vi "FTW-Test-JSON-Path.vi"() -> (0 "Test Result":errorcluster)   [LabVIEW 2015]
uses:
  src/json/FTW-JSON-Type.ctl
  src/json/core/FTW-JSON-Core-Type.ctl
  src/reflection/FTW-Reflection-Types.ctl
  src/json/core/FTW-JSON-Core-NumericType.vi
  lib/FTW-KernelFilepath.vi
  src/error/FTW-ERR-ThrowError.vi
  src/error/FTW-ERR-ThrowInvalidReferenceError.vi
  src/json/core/FTW-JSON-Core-ElementType.vi
  codegen/xnode/json/fetch/FTW-JSON-Core-GetFlattenedValue.vi
  codegen/xnode/FTW-JSON-Fetch.xnode
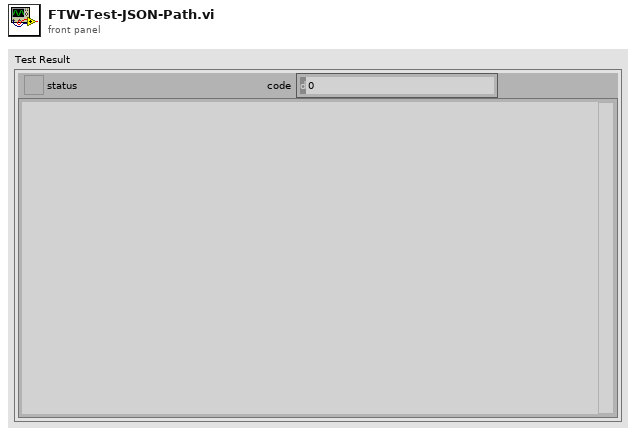
[diagram p1: front panel]
types:
  T1 = typedef "FTW-JSON-Type.ctl" = enum8{"Not Found", "Object", "Array", "String", "Number", "Boolean", "null"}
  T2 = cluster{"Path":string, "ExpectedValue":i32, "ExpectedType":T1}[]
  T3 = typedef "FTW-Type-JSON.ctl" = refnum<data-value>
  T4 = typedef "FTW-JSON-Core-Type.ctl" = enum8{"Object", "Array", "String", "Integer", "Floating Point", "true", "false", "null", "undefined"}
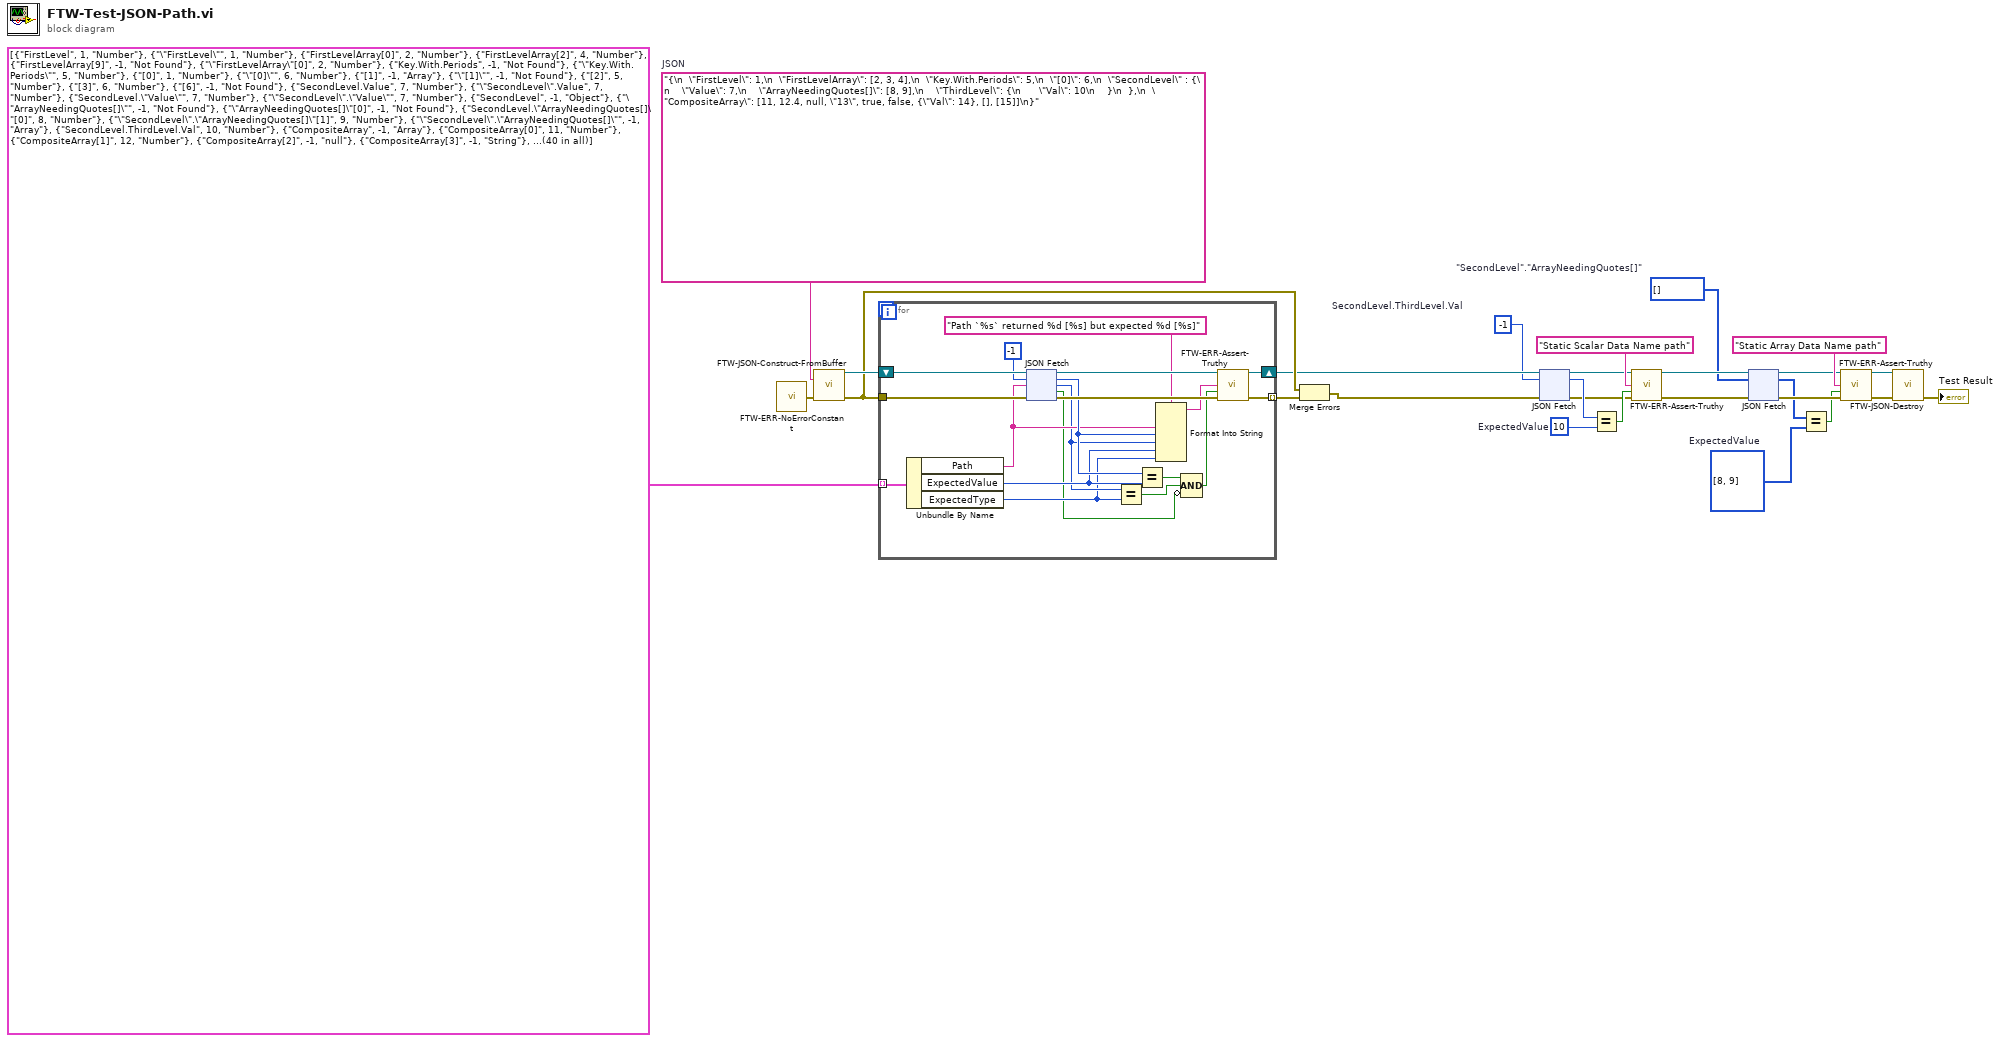
[diagram p0: block diagram]
diagram:
  w4 = i32[] [8, 9]  # ExpectedValue
  w2 = i32[] []  # "SecondLevel"."ArrayNeedingQuotes[]"
  w13 = 10  # ExpectedValue
  w3 = -1  # SecondLevel.ThirdLevel.Val
  w24 = "{\n  \"FirstLevel\": 1,\n  \"FirstLevelArray\": [2, 3, 4],\n  \"Key.With.Periods\": 5,\n  \"[0]\": 6,\n  \"SecondLevel\" : {\n    \"Value\": 7,\n    \"ArrayNeedingQuotes[]\": [8, 9],\n    \"ThirdLevel\": {\n      \"Val\": 10\n    }\n  },\n  \"CompositeArray\": [11, 12.4, null, \"13\", true, false, {\"Val\": 14}, [], [15]]\n}"  # JSON
  n1 = call "FTW-ERR-NoErrorConstant.vi"() -> ("no error"=w25:errorcluster)
  n2 = call "FTW-JSON-Construct-FromBuffer.vi"("JSON String (UTF-8)"=w24, "error in"=w25) -> ("JSON"=w23:T3, "error out"=w22:errorcluster)  [unwired: 12 in]
  n3 = for {
    tunnel: w22 -> [w43]
    tunnel: T2 [{"Path"="FirstLevel", "ExpectedValue"=1, "ExpectedType"=enum."Number"}, {"Path"="\"FirstLevel\"", "ExpectedValue"=1, "ExpectedType"=enum."Number"}, {"Path"="FirstLevelArray[0]", "ExpectedValue"=2, "ExpectedType"=enum."Number"}, {"Path"="FirstLevelArray[2]", "ExpectedValue"=4, "ExpectedType"=enum."Number"}, {"Path"="FirstLevelArray[9]", "ExpectedValue"=-1, "ExpectedType"=enum."Not Found"}, {"Path"="\"FirstLevelArray\"[0]", "ExpectedValue"=2, "ExpectedType"=enum."Number"}, {"Path"="Key.With.Periods", "ExpectedValue"=-1, "ExpectedType"=enum."Not Found"}, {"Path"="\"Key.With.Periods\"", "ExpectedValue"=5, "ExpectedType"=enum."Number"}, {"Path"="[0]", "ExpectedValue"=1, "ExpectedType"=enum."Number"}, {"Path"="\"[0]\"", "ExpectedValue"=6, "ExpectedType"=enum."Number"}, {"Path"="[1]", "ExpectedValue"=-1, "ExpectedType"=enum."Array"}, {"Path"="\"[1]\"", "ExpectedValue"=-1, "ExpectedType"=enum."Not Found"}, {"Path"="[2]", "ExpectedValue"=5, "ExpectedType"=enum."Number"}, {"Path"="[3]", "ExpectedValue"=6, "ExpectedType"=enum."Number"}, {"Path"="[6]", "ExpectedValue"=-1, "ExpectedType"=enum."Not Found"}, {"Path"="SecondLevel.Value", "ExpectedValue"=7, "ExpectedType"=enum."Number"}, {"Path"="\"SecondLevel\".Value", "ExpectedValue"=7, "ExpectedType"=enum."Number"}, {"Path"="SecondLevel.\"Value\"", "ExpectedValue"=7, "ExpectedType"=enum."Number"}, {"Path"="\"SecondLevel\".\"Value\"", "ExpectedValue"=7, "ExpectedType"=enum."Number"}, {"Path"="SecondLevel", "ExpectedValue"=-1, "ExpectedType"=enum."Object"}, {"Path"="\"ArrayNeedingQuotes[]\"", "ExpectedValue"=-1, "ExpectedType"=enum."Not Found"}, {"Path"="\"ArrayNeedingQuotes[]\"[0]", "ExpectedValue"=-1, "ExpectedType"=enum."Not Found"}, {"Path"="SecondLevel.\"ArrayNeedingQuotes[]\"[0]", "ExpectedValue"=8, "ExpectedType"=enum."Number"}, {"Path"="\"SecondLevel\".\"ArrayNeedingQuotes[]\"[1]", "ExpectedValue"=9, "ExpectedType"=enum."Number"}, {"Path"="\"SecondLevel\".\"ArrayNeedingQuotes[]\"", "ExpectedValue"=-1, "ExpectedType"=enum."Array"}, {"Path"="SecondLevel.ThirdLevel.Val", "ExpectedValue"=10, "ExpectedType"=enum."Number"}, {"Path"="CompositeArray", "ExpectedValue"=-1, "ExpectedType"=enum."Array"}, {"Path"="CompositeArray[0]", "ExpectedValue"=11, "ExpectedType"=enum."Number"}, {"Path"="CompositeArray[1]", "ExpectedValue"=12, "ExpectedType"=enum."Number"}, {"Path"="CompositeArray[2]", "ExpectedValue"=-1, "ExpectedType"=enum."null"}, {"Path"="CompositeArray[3]", "ExpectedValue"=-1, "ExpectedType"=enum."String"}, {"Path"="CompositeArray[4]", "ExpectedValue"=1, "ExpectedType"=enum."Boolean"}, {"Path"="CompositeArray[5]", "ExpectedValue"=0, "ExpectedType"=enum."Boolean"}, {"Path"="CompositeArray[6]", "ExpectedValue"=-1, "ExpectedType"=enum."Object"}, {"Path"="CompositeArray[6].Val", "ExpectedValue"=14, "ExpectedType"=enum."Number"}, {"Path"="CompositeArray[7]", "ExpectedValue"=-1, "ExpectedType"=enum."Array"}, {"Path"="CompositeArray[8][0]", "ExpectedValue"=15, "ExpectedType"=enum."Number"}, {"Path"="CompositeArray[8][1]", "ExpectedValue"=-1, "ExpectedType"=enum."Not Found"}, {"Path"="CompositeArray[9]", "ExpectedValue"=-1, "ExpectedType"=enum."Not Found"}, {"Path"="", "ExpectedValue"=-1, "ExpectedType"=enum."Object"}] -> [w42] mode=indexing
    shift-right: [w41] -> w19
    shift-left: w23 -> [w34]
    tunnel: [w38] -> w21 mode=indexing
    n4 = Unbundle By Name(w42) -> ("Path"=w33:string, "ExpectedValue"=w35:i32, "ExpectedType"=w27:T1)
    n5 = xnode "JSON Fetch"("JSON"=w34, "Element Type and Default Value"=-1, "Element Path"=w33, "error in"=w43) -> ("JSON out"=w41:T3, "Value"=w36:i32, "JSON Element Type"=w28:T1, "Consumed"=w26:bool, "error out"=w40:errorcluster)  [unwired: 1 in]
    n6 = Equal?(x=w28, y=w27) -> (x = y?=w30:bool)
    n7 = Equal?(x=w36, y=w35) -> (x = y?=w31:bool)
    n8 = Format Into String(format string="Path `%s` returned %d [%s] but expected %d [%s]" ("Assertion"), w33, w36, w28, w35, w27) -> (resulting string=w37:string)  [unwired: 2 in, 1 out]
    n9 = Compound Arithmetic op=AND(w31, w30, invert w26) -> (w29:bool)
    n10 = call "FTW-ERR-Assert-Truthy.vi"("Assertion"=w37, "Assertion holds true?"=w29, "error in"=w40) -> ("error out"=w38:errorcluster)  [unwired: 12 in]
  }
  n11 = Merge Errors(w22, w21) -> (w18:errorcluster)
  n12 = xnode "JSON Fetch"("JSON"=w19, "Element Type and Default Value"=w3, "error in"=w18) -> ("JSON out"=w8:T3, "Value"=w17:i32, "error out"=w15:errorcluster)  [unwired: 2 in, 2 out]
  n13 = Equal?(x=w17, y=w13) -> (x = y?=w16:bool)
  n14 = call "FTW-ERR-Assert-Truthy.vi"("Assertion"="Static Scalar Data Name path", "Assertion holds true?"=w16, "error in"=w15) -> ("error out"=w6:errorcluster)  [unwired: 12 in]
  n15 = xnode "JSON Fetch"("JSON"=w8, "Element Type and Default Value"=w2, "error in"=w6) -> ("JSON out"=w7:T3, "Value"=w9:i32[], "error out"=w11:errorcluster)  [unwired: 2 in, 2 out]
  n16 = Equal?(x=w9, y=w4) -> (x = y?=w10:bool)
  n17 = call "FTW-ERR-Assert-Truthy.vi"("Assertion"="Static Array Data Name path", "Assertion holds true?"=w10, "error in"=w11) -> ("error out"=w5:errorcluster)  [unwired: 12 in]
  n18 = call "FTW-JSON-Destroy.vi"("JSON"=w7, "error in"=w5) -> ("error out"=→"Test Result":errorcluster)  [unwired: 13 in]
